vi "PGA305.vi"() -> ()   [LabVIEW 2023]
panel:
  out "Read IC Serial number:":i32
  in  "ReadIcSerial?":bool
  in  "Serial number as integer":u64
  in  "WriteICSerial?":bool
  out "Write IC Serial status":string[](array[string])
  out "CRC":string
  out "Status":string
  in  "CRC":bool
  in  "Coefficients 2":string[](array[string])
  in  "Upload":bool
  out "Coefficients":string[](array[string])
  in  "Dac":dbl[](array[numeric]) format="%#.0f"
  in  "Tadc":dbl[](array[numeric]) format="%#.0f"
  in  "Coefficient":bool
  in  "Padc":dbl[](array[numeric]) format="%#.0f"
  in  "y":bool
  out "HEX":string
  in  "Multimeter USB port":refnum<visa-resource-name>
  in  "Activate OWI on Serial number":u16(ring) items=["445B9C6E17001A00"]
  in  "Set point":i32
  in  "Calibrate DAC":bool
  out "Waveform Chart 2":cluster{"[0]":dbl, "[1]":dbl}(graph)
  out "Padc & Tadc average":i32[](array[numeric])
  in  "Count":i32
  in  "Read ADC values":bool
  out "Waveform Chart":dbl(graph)
  out "Internal temperature sensor value":dbl
  in  "Read internal temp sensor":bool
  out "GPIO pin status":string
  in  "State":bool
  in  "GPIO pin":i16
  in  "Read? 2":bool
  out "Set additional voltage status":string
  in  "Voltage?":bool
  in  "Set Additional voltage (0-2v)":i8 min=0 max=2 step=1
  out "Rloop status":string
  in  "Rloop?":bool
  in  "Set Rloop ohm (0-50 ohm)":i8 min=0 max=50
  in  "Activate?":bool
  in  "Read?":bool
  in  "Write?":bool
  out "Read status":string[](array[string])
  in  "Read register":i16
  in  "Write register":i16
  in  "Read location":string[](array[string])
  in  "Write data":string[](array[string])
  out "Write status":string[](array[string])
  in  "Write location":string[](array[string])
  out "OWI Activate Status":string
  out "USB2ANY Firmware":string[](array[string])
  out "Connected to USB2ANY":string[](array[string])
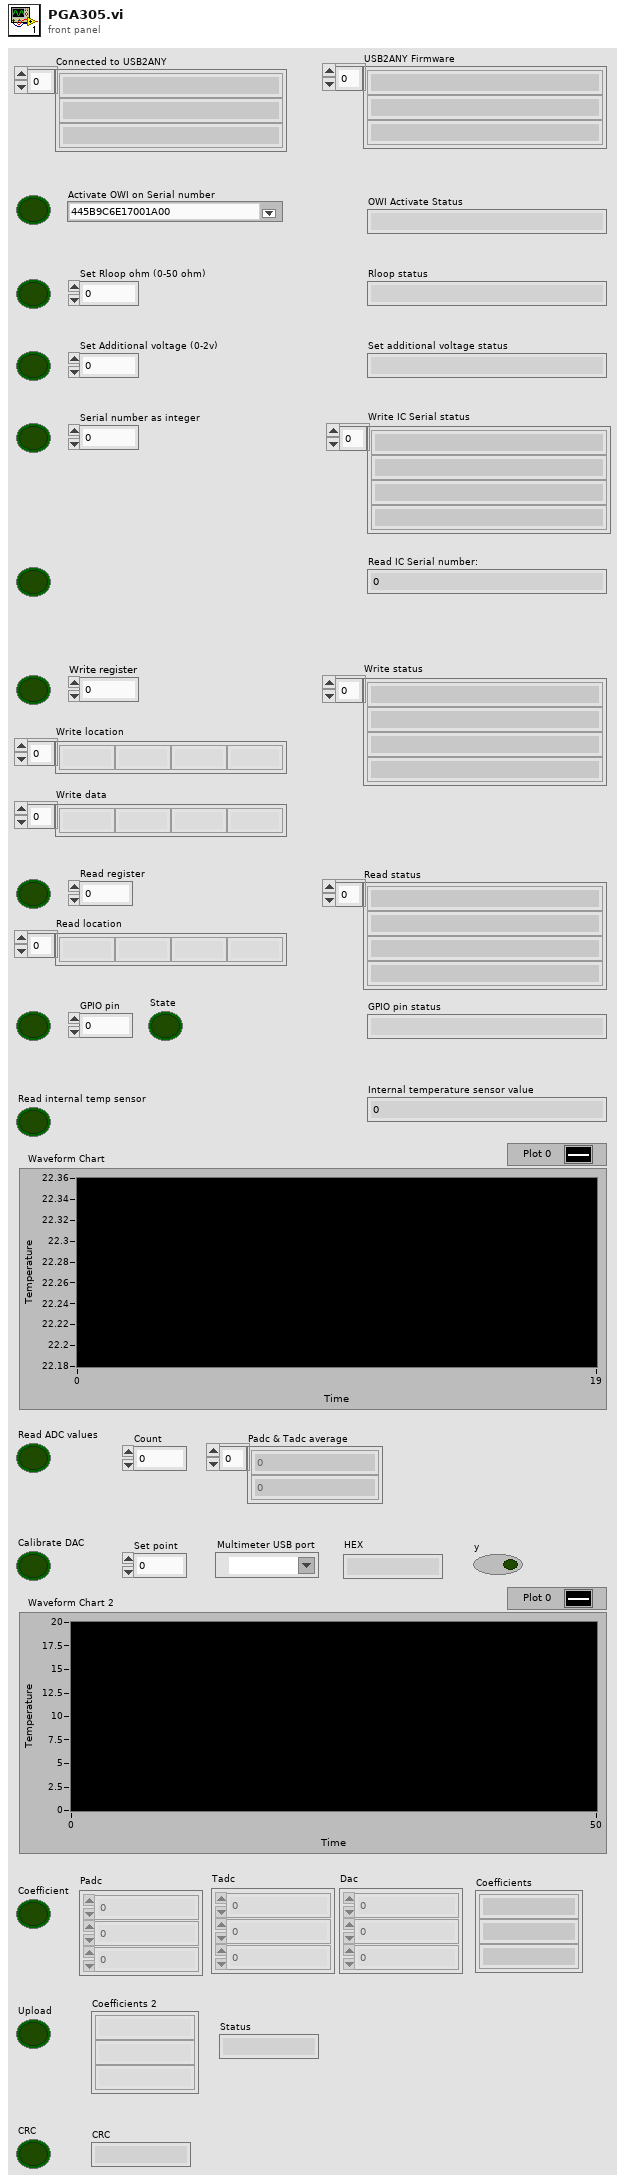
[diagram p1: front panel]
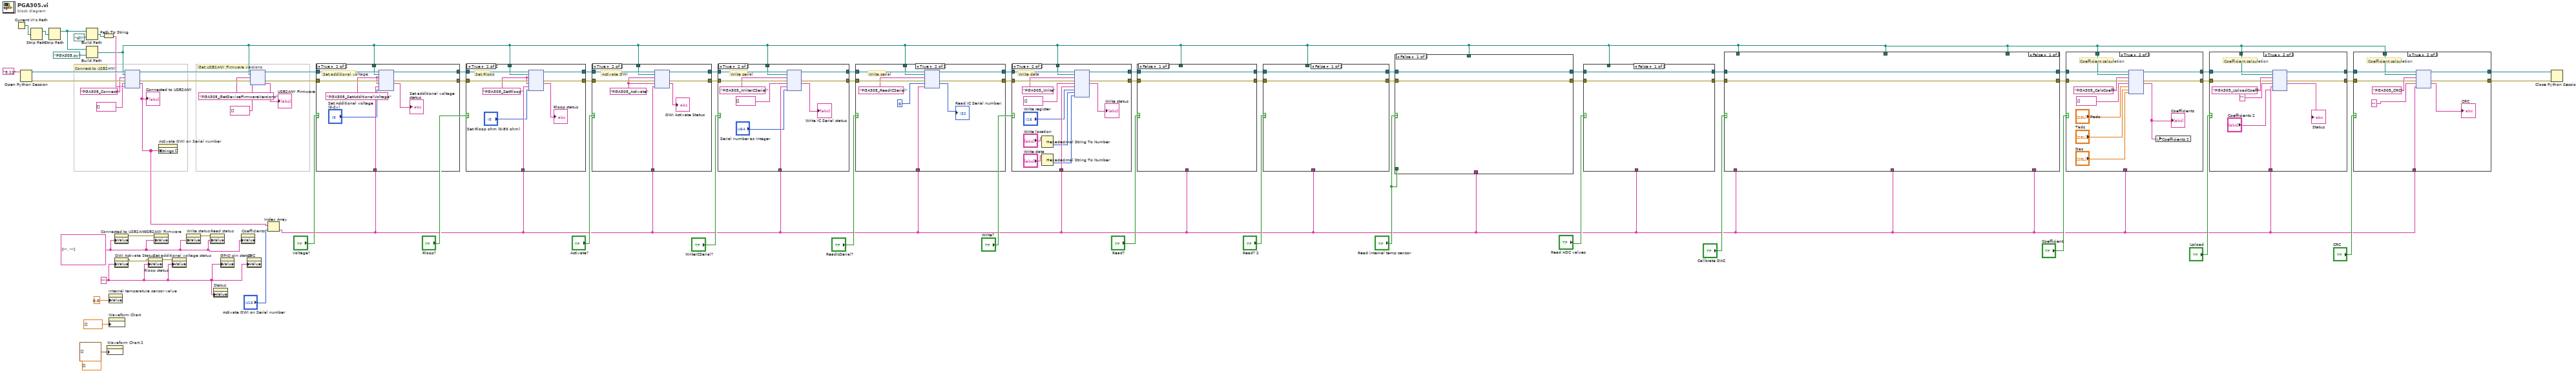
[diagram p0: block diagram]
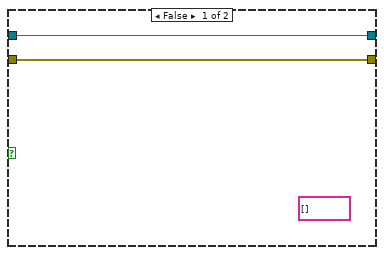
[diagram p6: hidden frame]
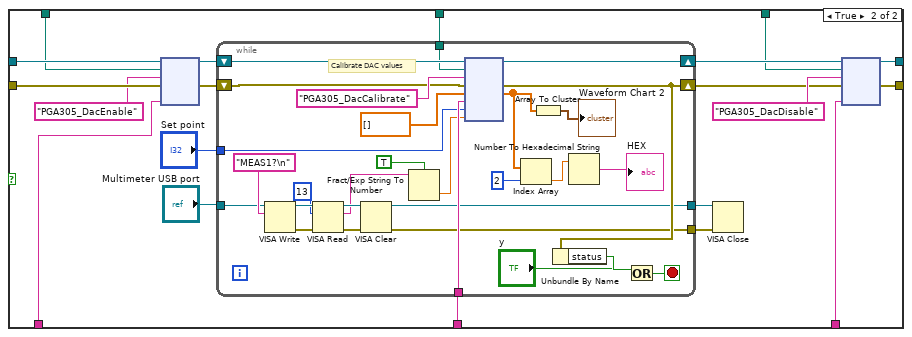
[diagram p7: hidden frame]
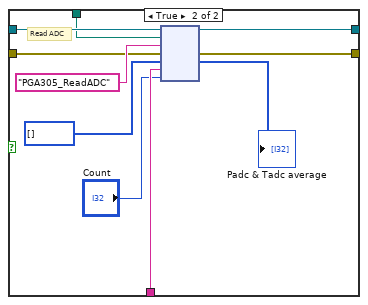
[diagram p8: hidden frame]
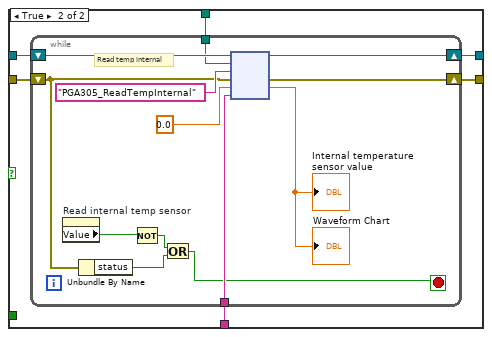
[diagram p9: hidden frame]
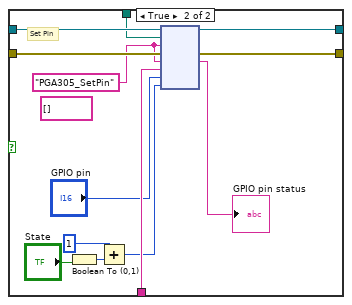
[diagram p10: hidden frame]
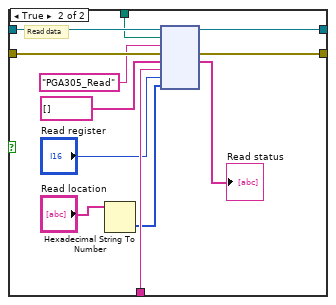
[diagram p14: hidden frame]
diagram:
  (unwired) dbl[] [] ("History Data")
  w11 = ""
  w12 = string[] ["", ""] ("Connected to USB2ANY")
  # "Get USB2ANY Firmware versions"
  # "Connect to USB2ANY"
  n1 = Current VI's Path() -> (path=w37:path)
  n2 = Open Python Session(python version="3.11" ("Python version")) -> (session out=w73:refnum<k35>, error out=w72:errorcluster)  [unwired: 2 in]
  n3 = Strip Path(path=w37) -> (stripped path=w36:path)  [unwired: 1 out]
  n4 = Strip Path(path=w36) -> (stripped path=w34:path)  [unwired: 1 out]
  n5 = Build Path(base path=w34, name or relative path=path "dll") -> (appended path=w35:path)
  n6 = Build Path(base path=w34, name or relative path=path "PGA305.py") -> (appended path=w2:path)
  n7 = Path To String(path=w35) -> (string=w69:string)
  n8 = property on="Waveform Chart 2" class="WFChart (strict)"("History Data"=cluster{"[0]":dbl, "[1]":dbl}[] []) -> ()  [unwired: 2 in, 2 out]
  n9 = property on="Internal temperature sensor value" class="DigNum (strict)"("Value"=0.0 ("Internal temperature sensor value")) -> ()  [unwired: 2 in, 2 out]
  n10 = property on="Waveform Chart" class="WFChart (strict)"("History Data"=dbl[] []) -> ()  [unwired: 2 in, 2 out]
  n11 = property on="Connected to USB2ANY" class="Arr (strict)"("Value"=w12) -> (error out=w58:errorcluster)  [unwired: 2 in, 1 out]
  n12 = property on="OWI Activate Status" class="Str"("Value"=w11) -> (error out=w47:errorcluster)  [unwired: 2 in, 1 out]
  n13 = node(w73, w2, "PGA305_Connect" ("function name"), w72, string[] [], w69) -> (w67:refnum<k35>, w66:errorcluster, w24:string[])  [unwired: 1 in, 2 out]
  "Connected to USB2ANY" <- w24
  n14 = property on="Rloop status" class="Str"(error in=w47, "Value"=w11) -> (error out=w46:errorcluster)  [unwired: 1 in, 1 out]
  n15 = property on="USB2ANY Firmware" class="Arr (strict)"(error in=w58, "Value"=w12) -> ()  [unwired: 1 in, 2 out]
  n16 = property on="Activate OWI on Serial number" class="Ring (strict)"("Strings []"=w24) -> ()  [unwired: 2 in, 2 out]
  n17 = property on="Set additional voltage status" class="Str"(error in=w46, "Value"=w11) -> ()  [unwired: 1 in, 2 out]
  n18 = property on="Write status" class="Arr (strict)"("Value"=w12) -> (error out=w57:errorcluster)  [unwired: 2 in, 1 out]
  n19 = property on="Read status" class="Arr (strict)"(error in=w57, "Value"=w12) -> ()  [unwired: 1 in, 2 out]
  n20 = property on="Status" class="Str"("Value"=w11) -> ()  [unwired: 2 in, 2 out]
  n21 = property on="GPIO pin status" class="Str"("Value"=w11) -> ()  [unwired: 2 in, 2 out]
  n22 = property on="Coefficients" class="Arr (strict)"("Value"=w12) -> ()  [unwired: 2 in, 2 out]
  n23 = property on="CRC" class="Str"("Value"=w11) -> ()  [unwired: 2 in, 2 out]
  n24 = node(w67, w2, "PGA305_GetDeviceFirmwareVersions" ("function name"), w66, string[] []) -> (w51:refnum<k35>, w50:errorcluster, →"USB2ANY Firmware":string[])  [unwired: 2 out]
  n25 = Index Array(array=w24, index="Activate OWI on Serial number") -> (element=w1:string)
  n26 = case shown="True" "Voltage?" {
    tunnel: [w76 w85] -> w49
    tunnel: [w75 w84] -> w48
    tunnel: w51 -> [w76 w83]
    tunnel: w50 -> [w75 w82]
    tunnel: w1 -> [_ w81]
    tunnel: w2 -> [_ w77]
    frame False {
    }
    frame True {
      w78 = "PGA305_SetAdditionalVoltage" ("function name")
      # "Set additional voltage"
      n27 = node(w83, w77, w78, w82, w78, w81, "Set Additional voltage (0-2v)") -> (w85:refnum<k35>, w84:errorcluster, →"Set additional voltage status":string)  [unwired: 2 in, 2 out]
    }
  }
  n28 = case shown="True" "Rloop?" {
    tunnel: [w87 w96] -> w55
    tunnel: [w86 w95] -> w54
    tunnel: w49 -> [w87 w94]
    tunnel: w48 -> [w86 w93]
    tunnel: w1 -> [_ w92]
    tunnel: w2 -> [_ w88]
    frame False {
    }
    frame True {
      w90 = "PGA305_SetRloop" ("function name")
      # "Set Rloop"
      n29 = node(w94, w88, w90, w93, w90, w92, "Set Rloop ohm (0-50 ohm)") -> (w96:refnum<k35>, w95:errorcluster, →"Rloop status":string)  [unwired: 2 in, 2 out]
    }
  }
  n30 = case shown="True" "Activate?" {
    tunnel: w55 -> [w98 w106]
    tunnel: w54 -> [w97 w105]
    tunnel: [w98 w102] -> w10
    tunnel: [w97 w101] -> w9
    tunnel: w1 -> [_ w100]
    tunnel: w2 -> [_ w99]
    frame False {
    }
    frame True {
      w104 = "PGA305_Activate" ("function name")
      # "Activate OWI"
      n31 = node(w106, w99, w104, w105, w104, w100) -> (w102:refnum<k35>, w101:errorcluster, →"OWI Activate Status":string)  [unwired: 1 in, 2 out]
    }
  }
  n32 = case shown="True" "WriteICSerial?" {
    tunnel: w10 -> [w108 w118]
    tunnel: w9 -> [w107 w117]
    tunnel: [w108 w113] -> w5
    tunnel: [w107 w112] -> w6
    tunnel: w1 -> [_ w111]
    tunnel: w2 -> [_ w109]
    frame False {
    }
    frame True {
      # "Write serial"
      n33 = node(w118, w109, "PGA305_WriteICSerial" ("function name"), w117, string[] [], w111, "Serial number as integer") -> (w113:refnum<k35>, w112:errorcluster, →"Write IC Serial status":string[])  [unwired: 2 in, 2 out]
    }
  }
  n34 = case shown="True" "ReadIcSerial?" {
    tunnel: w5 -> [w120 w129]
    tunnel: w6 -> [w119 w128]
    tunnel: [w120 w125] -> w4
    tunnel: [w119 w124] -> w3
    tunnel: w1 -> [_ w123]
    tunnel: w2 -> [_ w122]
    frame False {
    }
    frame True {
      # "Write serial"
      n35 = node(w129, w122, "PGA305_ReadICSerial" ("function name"), w128, 0, w123) -> (w125:refnum<k35>, w124:errorcluster, →"Read IC Serial number:":i32)  [unwired: 1 in, 2 out]
    }
  }
  n36 = case shown="True" "Write?" {
    tunnel: w4 -> [w131 w145]
    tunnel: w3 -> [w130 w144]
    tunnel: [w131 w140] -> w62
    tunnel: [w130 w139] -> w61
    tunnel: w1 -> [_ w138]
    tunnel: w2 -> [_ w132]
    frame False {
    }
    frame True {
      # "Write data"
      n37 = Hexadecimal String To Number(string="Write location") -> (number=w134:u32[])  [unwired: 2 in, 1 out]
      n38 = Hexadecimal String To Number(string="Write data") -> (number=w133:u32[])  [unwired: 2 in, 1 out]
      n39 = node(w145, w132, "PGA305_Write" ("function name"), w144, string[] [], w138, "Write register", w134, w133) -> (w140:refnum<k35>, w139:errorcluster, →"Write status":string[])  [unwired: 4 in, 2 out]
    }
  }
  n40 = case shown="False" "Read?" {
    tunnel: w62 -> [w147 w159]
    tunnel: w61 -> [w146 w158]
    tunnel: [w147 w157] -> w45
    tunnel: [w146 w156] -> w44
    tunnel: w1 -> [_ w154]
    tunnel: w2 -> [_ w148]
    frame False {
    }
    frame True {
      # "Read data"
      n41 = Hexadecimal String To Number(string="Read location") -> (number=w149:u32[])  [unwired: 2 in, 1 out]
      n42 = node(w159, w148, "PGA305_Read" ("function name"), w158, string[] [], w154, "Read register", w149) -> (w157:refnum<k35>, w156:errorcluster, →"Read status":string[])  [unwired: 3 in, 2 out]
    }
  }
  n43 = case shown="False" "Read? 2" {
    tunnel: [w161 w169] -> w42
    tunnel: [w160 w168] -> w41
    tunnel: w45 -> [w161 w174]
    tunnel: w44 -> [w160 w173]
    tunnel: w1 -> [_ w172]
    tunnel: w2 -> [_ w162]
    frame False {
    }
    frame True {
      (unwired) string[] []
      w164 = "PGA305_SetPin" ("function name")
      # "Set Pin"
      n44 = Boolean To (0,1)(Boolean="State") -> (0, 1=w167:i16)
      n45 = Add(x=i16 1, y=w167) -> (x+y=w165:i16)
      n46 = node(w174, w162, w164, w173, w164, w172, "GPIO pin", w165) -> (w169:refnum<k35>, w168:errorcluster, →"GPIO pin status":string)  [unwired: 3 in, 2 out]
    }
  }
  n47 = case shown="False" "Read internal temp sensor" {
    tunnel: [w176 w181] -> w32
    tunnel: [w175 w182] -> w31
    tunnel: w42 -> [w176 w180]
    tunnel: w41 -> [w175 w179]
    tunnel: w1 -> [_ w178]
    tunnel: "Read internal temp sensor" -> [_ _]
    tunnel: w2 -> [_ w177]
    frame False {
    }
    frame True {
      n48 = while {
        tunnel: w178 -> [w190]
        shift-right: [w193] -> w181
        shift-left: w180 -> [w192]
        shift-right: [w195] -> w182
        shift-left: w179 -> [w188]
        tunnel: w177 -> [w183]
        stop <- w186 stop-if-true
        # "Read temp internal"
        n49 = property on="Read internal temp sensor" class="Bool (strict)"() -> ("Value"=w184:bool)  [unwired: 2 in, 2 out]
        n50 = Unbundle By Name(w188) -> ("status"=w187:bool)
        n51 = Not(x=w184) -> (.not. x?=w185:bool)
        n52 = Or(x=w185, y=w187) -> (x .or. y?=w186:bool)
        n53 = node(w192, w183, "PGA305_ReadTempInternal" ("function name"), w188, 0.0, w190) -> (w193:refnum<k35>, w195:errorcluster, →"Internal temperature sensor value" →"Waveform Chart":dbl)  [unwired: 1 in, 2 out]
      }
    }
  }
  n54 = case shown="False" "Read ADC values" {
    tunnel: [w197 w206] -> w29
    tunnel: [w196 w205] -> w28
    tunnel: w32 -> [w197 w207]
    tunnel: w31 -> [w196 w203]
    tunnel: w2 -> [_ w202]
    tunnel: w1 -> [_ w201]
    frame False {
    }
    frame True {
      # "Read ADC"
      n55 = node(w207, w202, "PGA305_ReadADC" ("function name"), w203, i32[] [], w201, "Count") -> (w206:refnum<k35>, w205:errorcluster, →"Padc & Tadc average":i32[])  [unwired: 2 in, 2 out]
    }
  }
  n56 = case shown="False" "Calibrate DAC" {
    tunnel: [w209 w220] -> w23
    tunnel: [w208 w216] -> w22
    tunnel: w29 -> [w209 w227]
    tunnel: w28 -> [w208 w226]
    tunnel: w1 -> [_ w229]
    tunnel: w2 -> [_ w228]
    tunnel: w2 -> [_ w225]
    tunnel: w1 -> [_ w223]
    tunnel: w2 -> [_ w218]
    tunnel: w1 -> [_ w215]
    frame False {
    }
    frame True {
      n57 = node(w227, w225, "PGA305_DacEnable" ("function name"), w226, w223) -> (w222:refnum<k35>, w221:errorcluster)  [unwired: 3 in, 2 out]
      n58 = while {
        tunnel: w229 -> [w255]
        shift-right: [w257] -> w219
        shift-left: w222 -> [w256]
        shift-right: [w249] -> w213
        shift-left: w221 -> [w250]
        tunnel: w228 -> [w254]
        tunnel: "Set point" -> [w252]
        tunnel: "Multimeter USB port" -> [w244]
        tunnel: [w243] -> w211
        tunnel: [w233] -> w210
        stop <- w232 stop-if-true
        # "Calibrate DAC values"
        n59 = VISA Write(VISA resource name=w244, write buffer="MEAS1?\n") -> (VISA resource name out=w236:refnum<visa-resource-name>, error out=w235:errorcluster)  [unwired: 1 in, 1 out]
        n60 = VISA Read(VISA resource name=w236, byte count=u32 13, error in (no error)=w235) -> (VISA resource name out=w247:refnum<visa-resource-name>, read buffer=w242:string, error out=w248:errorcluster)  [unwired: 1 out]
        n61 = VISA Clear(VISA resource name=w247, error in (no error)=w248) -> (VISA resource name out=w243:refnum<visa-resource-name>, error out=w233:errorcluster)
        n62 = Fract/Exp String To Number(use system decimal point (T)=TRUE, string=w242) -> (number=w245:dbl)  [unwired: 2 in, 1 out]
        n63 = node(w256, w254, "PGA305_DacCalibrate" ("function name"), w250, dbl[] [], w255, w252, w245) -> (w257:refnum<k35>, w249:errorcluster, w238:dbl[])  [unwired: 3 in, 2 out]
        n64 = Index Array(array=w238, index=2) -> (element=w240:dbl)
        n65 = Array To Cluster(array=w238) -> (cluster=→"Waveform Chart 2":cluster{"[0]":dbl, "[1]":dbl})
        n66 = Unbundle By Name(w249) -> ("status"=w231:bool)
        n67 = Number To Hexadecimal String(2:w240) -> (0:→"HEX":string)  [unwired: 1 in]
        n68 = Or(x=w231, y="y") -> (x .or. y?=w232:bool)
      }
      n69 = VISA Close(VISA resource name=w211, error in (no error)=w210) -> ()  [unwired: 1 out]
      n70 = node(w219, w218, "PGA305_DacDisable" ("function name"), w213, w215) -> (w220:refnum<k35>, w216:errorcluster)  [unwired: 3 in, 2 out]
    }
  }
  n71 = case shown="True" "Coefficient" {
    tunnel: [w260 w270] -> w20
    tunnel: [w259 w269] -> w19
    tunnel: w23 -> [w260 w271]
    tunnel: w22 -> [w259 w267]
    tunnel: w2 -> [_ w266]
    tunnel: w1 -> [_ _]
    frame False {
      (unwired) string[] []
    }
    frame True {
      # "Coefficient calculation"
      n72 = node(w271, w266, "PGA305_CalcCoeff" ("function name"), w267, string[] [], "Padc", "Tadc", "Dac") -> (w270:refnum<k35>, w269:errorcluster, w261:string[])  [unwired: 3 in, 2 out]
      "Coefficients" <- w261
      n73 = local write "Coefficients 2"(w261) -> ()
    }
  }
  n74 = case shown="True" "Upload" {
    tunnel: [w273 w282] -> w17
    tunnel: [w272 w281] -> w16
    tunnel: w20 -> [w273 w283]
    tunnel: w19 -> [w272 w279]
    tunnel: w2 -> [_ w278]
    tunnel: w1 -> [_ w277]
    frame False {
    }
    frame True {
      # "Coefficient calculation"
      n75 = node(w283, w278, "PGA305_UploadCoeff" ("function name"), w279, "", w277, "Coefficients 2") -> (w282:refnum<k35>, w281:errorcluster, →"Status":string)  [unwired: 2 in, 2 out]
    }
  }
  n76 = case shown="True" "CRC" {
    tunnel: [w285 w293] -> w15
    tunnel: [w284 w292] -> w14
    tunnel: w17 -> [w285 w294]
    tunnel: w16 -> [w284 w290]
    tunnel: w2 -> [_ w289]
    tunnel: w1 -> [_ w288]
    frame False {
    }
    frame True {
      # "Coefficient calculation"
      n77 = node(w294, w289, "PGA305_CRC" ("function name"), w290, "", w288) -> (w293:refnum<k35>, w292:errorcluster, →"CRC":string)  [unwired: 1 in, 2 out]
    }
  }
  n78 = Close Python Session(session in=w15, error in=w14) -> ()  [unwired: 1 out]
